vi "CRYReport Function LIB.vi"(7 "sAction":string, 8 "nData":i32, 9 "sData":string, 10 "cView":T2, 11 "cFrame":T1) -> (0 "nData_Out":i32, 1 "sData_Out":string, 2 "cView_Out":T2, 3 "cFrame_Out":T1)   [LabVIEW 2013]
uses:
  CRYReport Global.vi
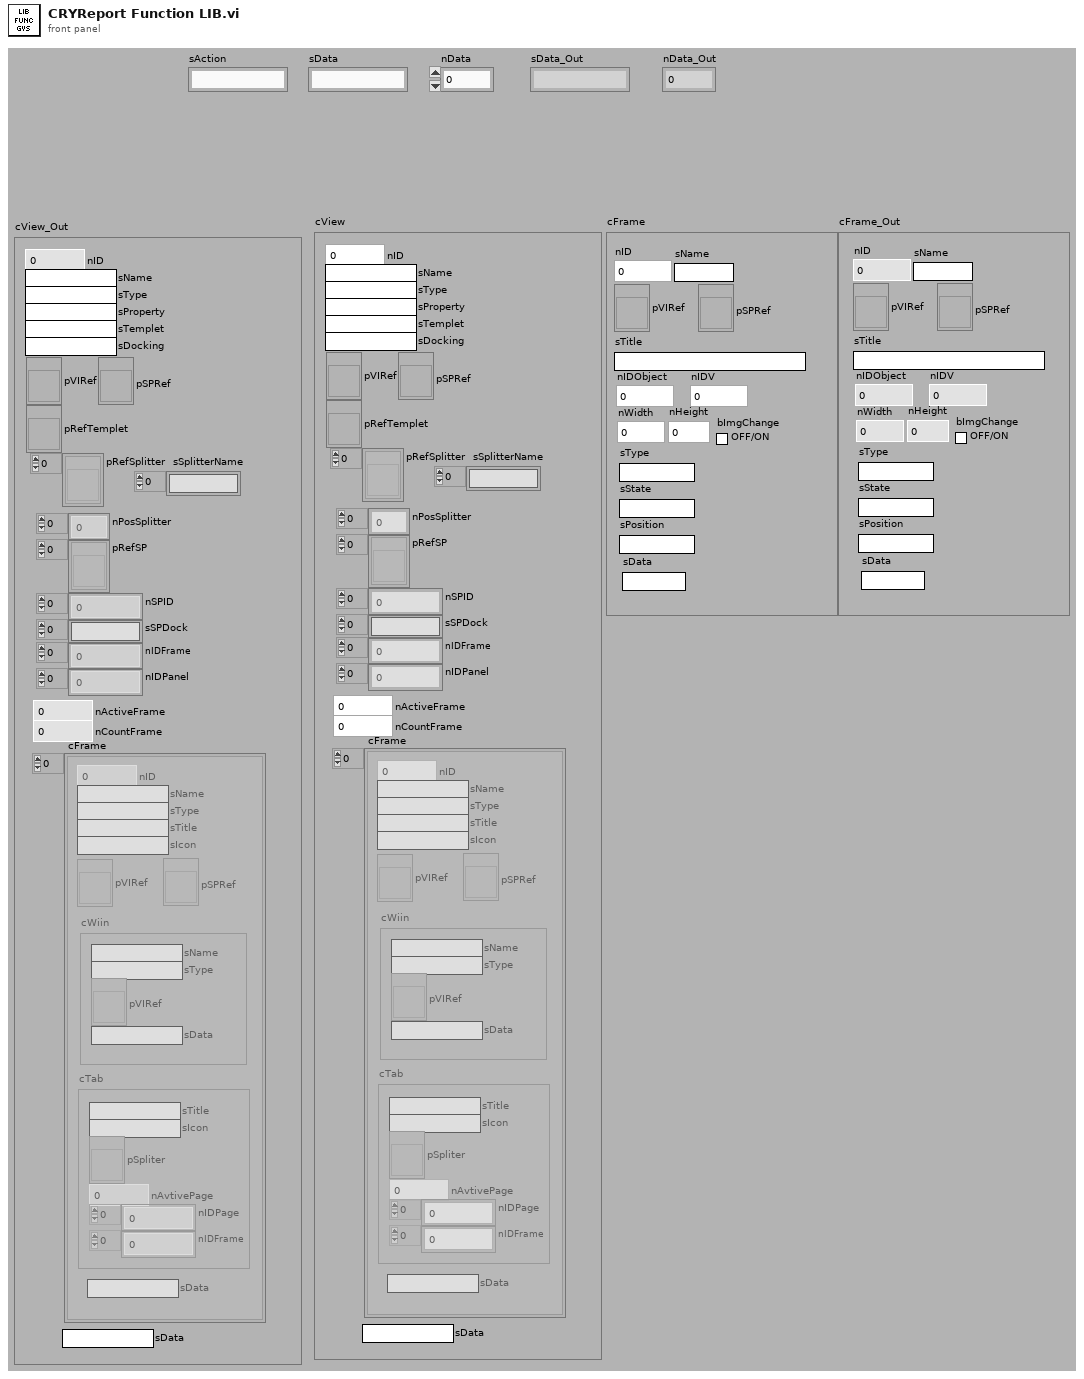
[diagram p1: front panel]
types:
  T1 = cluster{"nID":i16, "sName":string, "pVIRef":refnum<vi>, "pSPRef":refnum<vi>, "sTitle":string, "nIDObject":i16, "nIDV":i16, "nWidth":i16, "nHeight":i16, "bImgChange":bool, "sType":string, "sState":string, "sPosition":string, "sData":string}
  T2 = cluster{"nID":i32, "sName":string, "sType":string, "sProperty":string, "sTemplet":string, "sDocking":string, "pVIRef":refnum<vi>, "pSPRef":refnum<vi>, "pRefTemplet":refnum<vi>, "pRefSplitter":refnum<vi>[], "nPosSplitter":i32[], "pRefSP":refnum<vi>[], "nSPID":i32[], "sSPDock":string[], "nIDFrame":i32[], "nIDPanel":i32[], "nActiveFrame":i32, "nCountFrame":i32, "cFrame":cluster{"nID":i32, "sName":string, "sType":string, "sTitle":string, "sIcon":string, "pVIRef":refnum<vi>, "pSPRef":refnum<vi>, "cWiin":cluster{"sName":string, "sType":string, "pVIRef":refnum<vi>, "sData":string}, "cTab":cluster{"sTitle":string, "sIcon":string, "pSpliter":refnum<vi>, "nAvtivePage":i32, "nIDPage":i32[], "nIDFrame":i32[]}, "sData":string}[], "sData":string, "sSplitterName":string[]}
  T3 = cluster{"nCount":i16, "cFrameList":cluster{"nID":i16, "sName":string, "pVIRef":refnum<vi>, "pSPRef":refnum<vi>, "sTitle":string, "nIDObject":i16, "nIDV":i16, "nWidth":i16, "nHeight":i16, "bImgChange":bool, "sType":string, "sState":string, "sPosition":string, "sData":string}[], "sData":string}
  T4 = cluster{"nID":i16, "sName":string, "pVIRef":refnum<vi>, "pSPRef":refnum<vi>, "sTitle":string, "nIDObject":i16, "nIDV":i16, "nWidth":i16, "nHeight":i16, "bImgChange":bool, "sType":string, "sState":string, "sPosition":string, "sData":string}[]
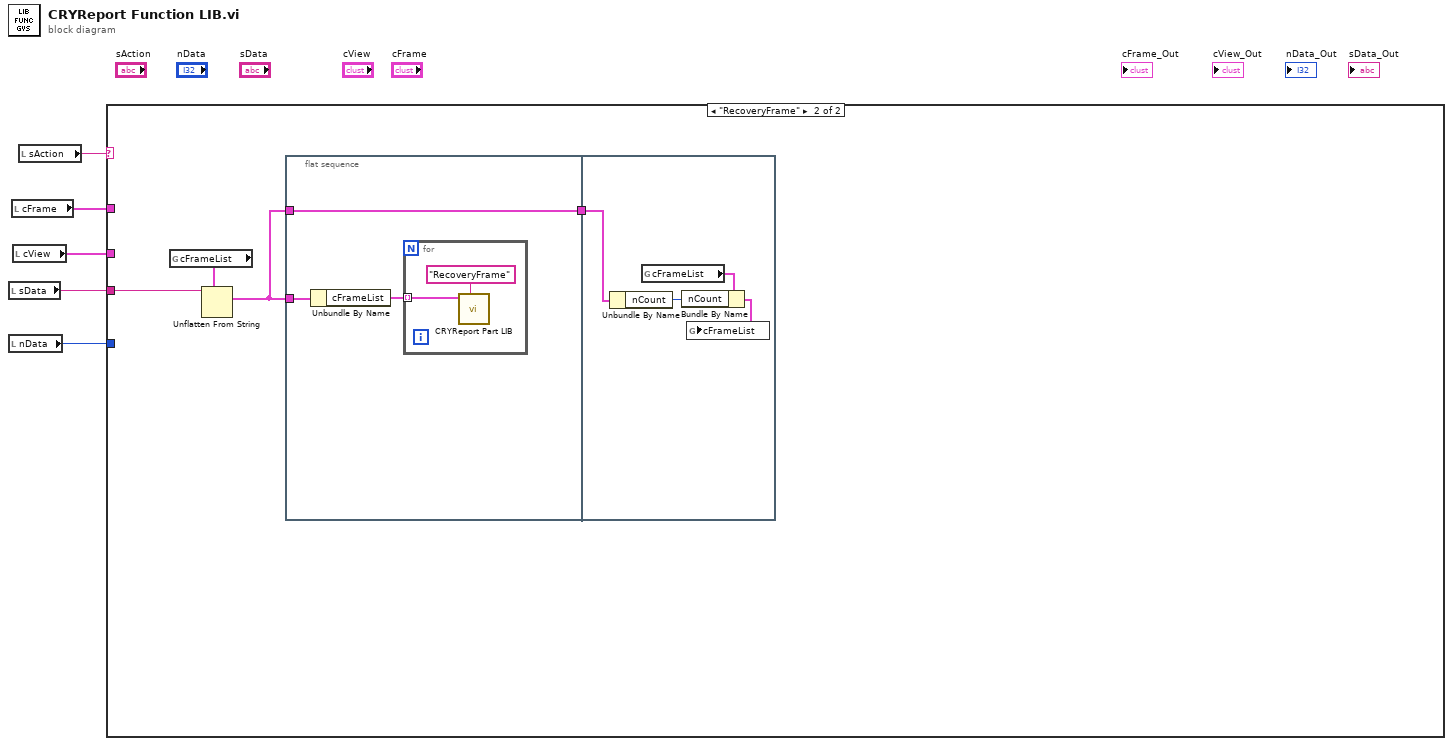
[diagram p0: block diagram]
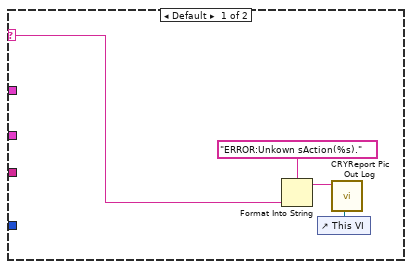
[diagram p2: hidden frame]
diagram:
  n1 = local read "sData"() -> (w4:string)
  n2 = local read "nData"() -> (w3:i32)
  n3 = local read "cFrame"() -> (w2:T1)
  n4 = local read "cView"() -> (w1:T2)
  n5 = local read "sAction"() -> (w5:string)
  n6 = case shown="\"RecoveryFrame\"" w5 {
    selector: w5 -> [w7 _]
    tunnel: w4 -> [_ w10]
    tunnel: w3 -> [_ _]
    tunnel: w2 -> [_ _]
    tunnel: w1 -> [_ _]
    frame Default {
      n7 = Format Into String(format string="ERROR:Unkown sAction(%s).", w7) -> (resulting string=w6:string)  [unwired: 2 in, 1 out]
      n8 = control-ref of="This VI"() -> (w9:refnum<vi>)
      n9 = call "CRYReport Pic Out Log.vi"("vi reference"=w9, "sData"=w6) -> ()  [unwired: 10 in]
    }
    frame "RecoveryFrame" {
      n10 = global read "CRYReport Global.vi" "cFrameList"() -> (w13:T3)
      n11 = Unflatten From String(type=w13, binary string=w10) -> (value=w11:T3)  [unwired: 3 in, 2 out]
      n12 = flat-sequence {
        tunnel: w11 -> [w16]
        tunnel: [w15] -> w12
        tunnel: w11 -> [w15]
        tunnel: w12 -> [w21]
        frame #0 {
          n13 = Unbundle By Name(w16) -> ("cFrameList"=w14:T4)
          n14 = for {
            tunnel: w14 -> [w17] mode=indexing
            n15 = call "CRYReport Part LIB.vi"("sAction"="RecoveryFrame", "cFrame"=w17) -> ()  [unwired: 6 in, 4 out]
          }
        }
        frame #1 {
          n16 = Unbundle By Name(w21) -> ("nCount"=w20:i16)
          n17 = global read "CRYReport Global.vi" "cFrameList"() -> (w22:T3)
          n18 = Bundle By Name(cluster=w22, "nCount"=w20) -> (w19:T3)
          n19 = global write "CRYReport Global.vi" "cFrameList"(w19) -> ()
        }
      }
    }
  }
